vi "ResetFPlocns.vi"() -> ()   [LabVIEW 2021]
panel:
  out "error IO":errorcluster
  # "Reset FP Locations"
  # "Reads in a file of your choosing and applies the Front Panel locations stored therein"
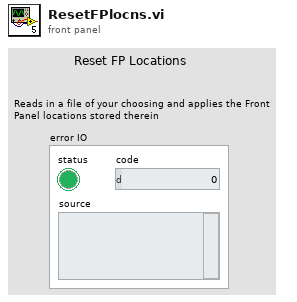
[diagram p1: front panel]
types:
  T1 = typedef "VInameSizePath.ctl" = cluster{"VI Name":string, "Front Panel.WinBounds":T2, "File Path":path}
  T2 = typedef "LVRectTypeDef.ctl" = cluster{"Left":i16, "Top":i16, "Right":i16, "Bottom":i16}
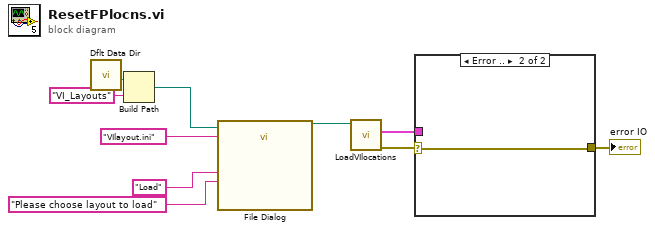
[diagram p0: block diagram]
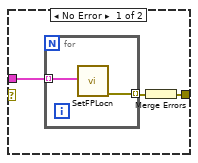
[diagram p2: hidden frame]
diagram:
  n1 = call <vilib>:"Dflt Data Dir.vi"() -> ("App:Default Data Directory"=w5:path)
  n2 = Build Path(base path=w5, name or relative path="VI_Layouts") -> (appended path=w6:path)
  n3 = call "File Dialog"("start path"=w6, "prompt"="Please choose layout to load", "button label"="Load", "default name"="VIlayout.ini") -> ("selected path"=w4:path)  [unwired: 8 in, 3 out]
  n4 = call "LoadVIlocations.vi"("configuration file path"=w4) -> ("error out"=w2:errorcluster, "NamesAndLocnsArray"=w10:T1[])  [unwired: 9 in]
  n5 = case shown="Error .." w2 {
    selector: w2 -> [_ w16]
    tunnel: w10 -> [w13 _]
    tunnel: [w11 w16] -> w1
    frame No Error {
      n6 = for {
        tunnel: w13 -> [w15] mode=indexing
        tunnel: [w14] -> w12 mode=indexing
        n7 = call "SetFPLocn.vi"("Cluster"=w15) -> ("error out"=w14:errorcluster)  [unwired: 10 in]
      }
      n8 = Merge Errors(w12) -> (w11:errorcluster)
    }
    frame Error {
    }
  }
  "error IO" <- w1
